vi "lib String to Array of Strings.vi"(8 "error in (no error)":errorcluster, 11 "Multi-line String":string) -> (0 "error out":errorcluster, 3 "Array":string[](array[string]))   [LabVIEW 2016]
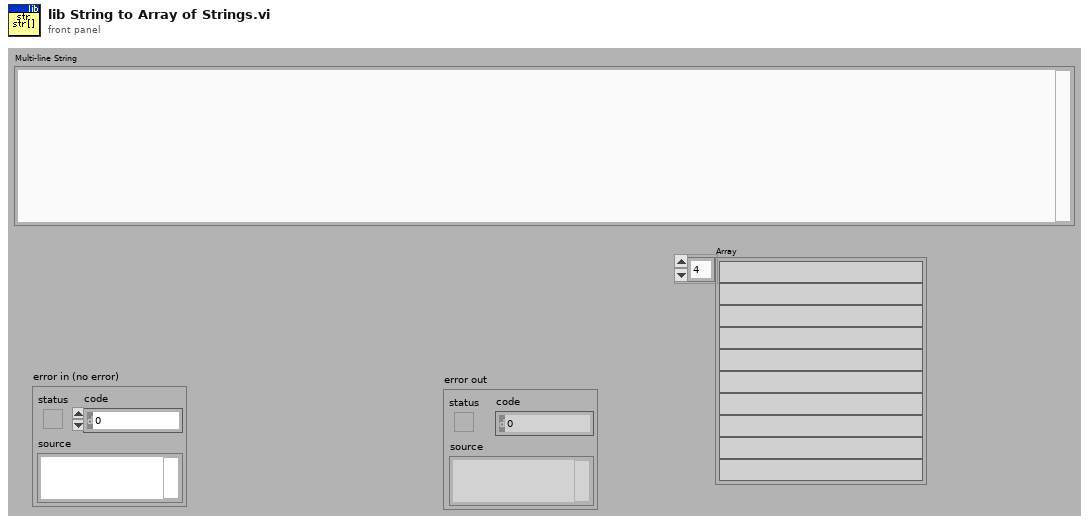
[diagram p1: front panel]
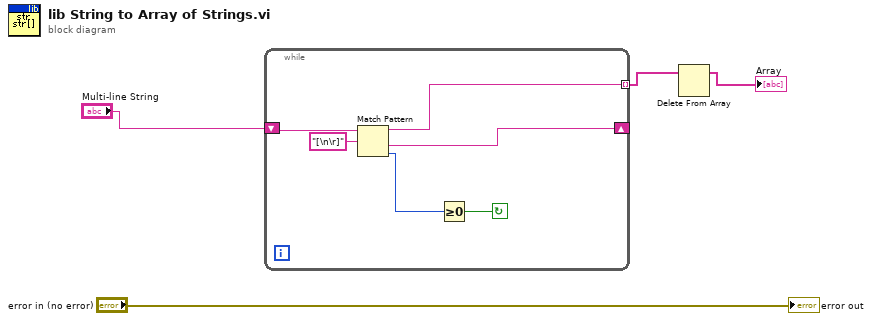
[diagram p0: block diagram]
diagram:
  n1 = while {
    shift-right: [w7] -> _
    shift-left: "Multi-line String" -> [w10]
    tunnel: [w8] -> w2 mode=indexing
    stop <- w5 continue-if-true
    n2 = Match Pattern(string=w10, regular expression="[\n\r]") -> (before substring=w8:string, after substring=w7:string, offset past match=w6:i32)  [unwired: 1 in, 1 out]
    n3 = Greater Or Equal To 0?(x=w6) -> (x >= 0?=w5:bool)
  }
  n4 = Delete From Array(array=w2) -> (array with subset deleted=→"Array":string[])  [unwired: 2 in, 1 out]
  "error out" <- "error in (no error)"
